vi "test-001.vi"() -> ()   [LabVIEW 2019]
uses:
  <vilib>/Platform/TimedLoop/XDataNode/timing_clust.ctl
  <vilib>/Platform/TimedLoop/XDataNode/nitl_modes.ctl
  <vilib>/Platform/TimedLoop/XDataNode/wakeup.ctl
  <vilib>/platform/TimedLoop/XDataNode/XDataNode.xnode
  <vilib>/Platform/TimedLoop/XDataNode/XDNodeRunTimeDep.lvlib
  <vilib>/ptbypt/NI_PtbyPt.lvlib
panel:
  in  "Stop":bool
  out "Waveform Chart":T1(graph)
  in  "D":dbl
  in  "J":dbl
  in  "A":dbl
  in  "V":dbl
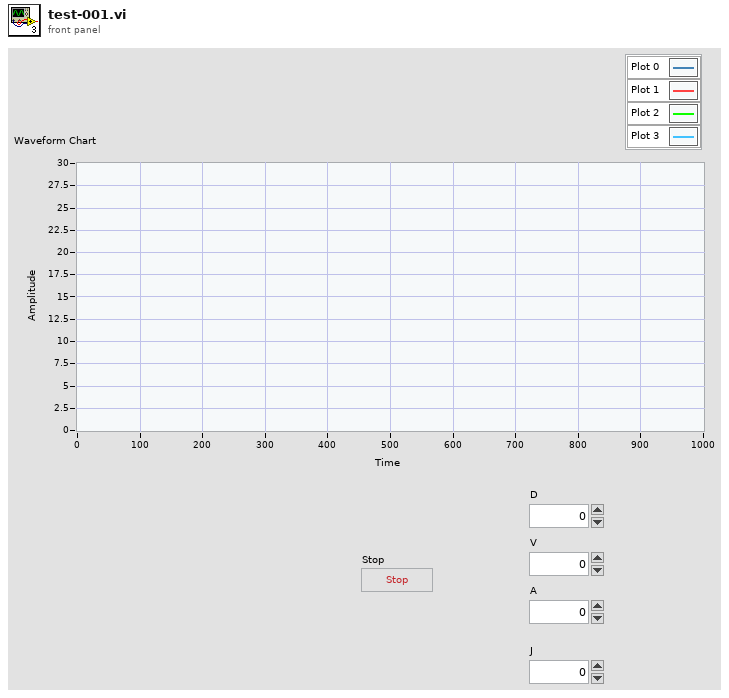
[diagram p1: front panel]
types:
  T1 = cluster{"setpoint":dbl, "integral x(t)":dbl, "integral x(t)":dbl, "integral x(t)":dbl}
  T2 = typedef "XDNodeRunTimeDep.lvlib/timing_clust.ctl" = cluster{"Expected End [f-1]":u64, "Actual End [f-1]":u64, "Finished Late? [f-1]":bool, "Expected End [i-1]":u64, "Actual End [i-1]":u64, "Finished Late? [i-1]":bool, "Expected Start [i]":u64, "Actual Start [i]":u64, "Expected Start [f]":u64, "Actual Start [f]":u64, "Source Name":string, "Structure Name":string, "Period":i64, "Deadline":i64, "Offset":i64, "Start":i64, "Priority":i32, "Timeout":i32, "Mode":T3, "Wakeup Reason":T4, "Error":errorcluster, "Source Type":string, "Secondary Source Type":string, "Global End Time":u64, "Global Start Time":u64, "Frame Duration":u64, "Iteration Duration":u64, "Assigned CPU":i32, "I/O Scan Engine Mode":u32}
  T3 = typedef "XDNodeRunTimeDep.lvlib/nitl_modes.ctl" = enum32{"No Change", "Process missed periods, maintain original phase", "Discard missed periods, maintain original phase", "Process missed periods, ignore original phase", "Discard missed periods, ignore original phase"}
  T4 = typedef "XDNodeRunTimeDep.lvlib/wakeup.ctl" = enum32{"Normal", "Aborted", "Asynchronous wakeup", "Timing source error", "Timed loop error", "Timeout"}
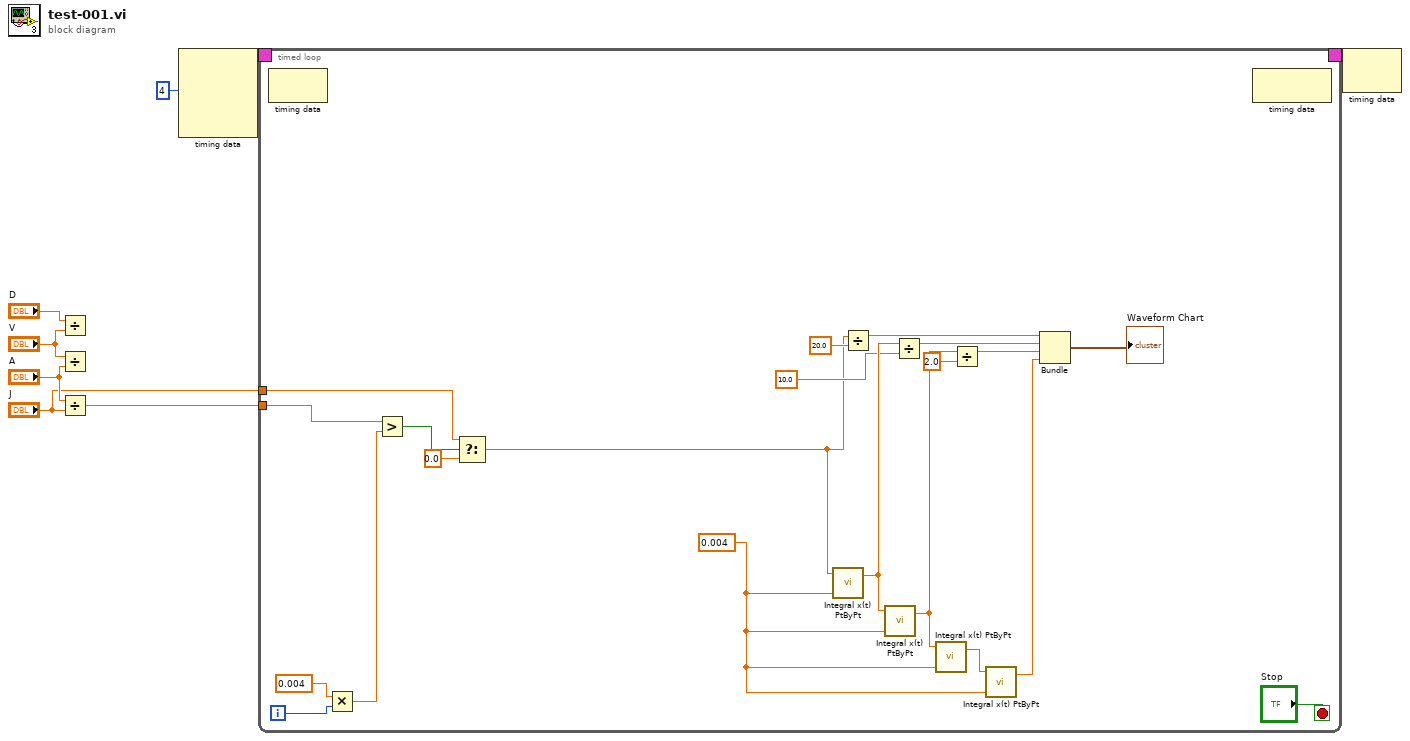
[diagram p0: block diagram]
diagram:
  n1 = Divide(x="D", y="V") -> ()  [unwired: 1 out]
  n2 = Divide(x="V", y="A") -> ()  [unwired: 1 out]
  n3 = Divide(x="A", y="J") -> (x/y=w3:dbl)
  n4 = node-c288(i64 4 ("Period")) -> (w7:T2)  [unwired: 3 in]
  n5 = timed-loop {
    timing: w7 -> [_]
    timing-out: [_] -> w6
    tunnel: w3 -> [w17]
    tunnel: "J" -> [w12]
    i -> [w15]
    stop <- "Stop" stop-if-true
    w26 = 0.004 ("dt (s)")
    n6 = node-c288() -> ()  [unwired: 1 in, 1 out]
    n7 = Multiply(x=0.004, y=w15) -> (x*y=w14:dbl)
    n8 = Greater?(x=w17, y=w14) -> (0:w13:bool)
    n9 = Select(t=w12, s=w13, f=0.0) -> (s? t:f=w9:dbl)
    n10 = call <vilib>:"Integral x(t) PtByPt.vi"("dt"=w26, "x"=w9) -> ("integral x(t)"=w29:dbl)  [unwired: 2 in, 1 out]
    n11 = Divide(x=w9, y=20.0) -> (x/y=w23:dbl)
    n12 = call <vilib>:"Integral x(t) PtByPt.vi"("dt"=w26, "x"=w29) -> ("integral x(t)"=w28:dbl)  [unwired: 2 in, 1 out]
    n13 = Divide(x=w29, y=10.0) -> (x/y=w21:dbl)
    n14 = call <vilib>:"Integral x(t) PtByPt.vi"("dt"=w26, "x"=w28) -> ("integral x(t)"=w27:dbl)  [unwired: 2 in, 1 out]
    n15 = Divide(x=w28, y=2.0) -> (x/y=w19:dbl)
    n16 = call <vilib>:"Integral x(t) PtByPt.vi"("dt"=w26, "x"=w27) -> ("integral x(t)"=w25:dbl)  [unwired: 2 in, 1 out]
    n17 = Bundle(w23, w21, w19, "integral x(t)"=w25) -> (→"Waveform Chart":cluster{dbl, dbl, dbl, "integral x(t)":dbl})  [unwired: 1 in]
    n18 = node-c288() -> ()  [unwired: 1 in, 1 out]
  }
  n19 = node-c288(w6) -> ()  [unwired: 1 out]
